vi "Init.vi"(8 "error in":errorcluster, 11 "IController in":refnum<class "IController.lvclass">) -> (0 "error out":errorcluster, 3 "IController out":refnum<class "IController.lvclass">)   [LabVIEW 2023, in "SourceGrid.lvlib" / "IController.lvclass"]
uses:
  IController.lvclass
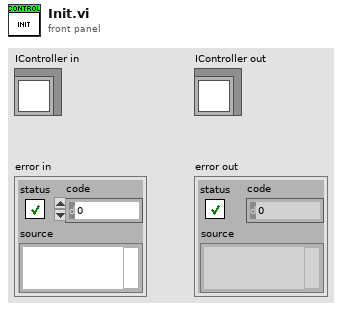
[diagram p1: front panel]
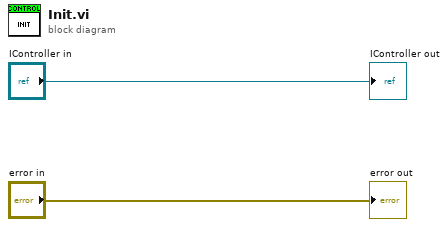
[diagram p0: block diagram]
diagram:
  "error out" <- "error in"
  "IController out" <- "IController in"
